vi "FindRequestBySummary.vi"(8 "error in (no error)":errorcluster, 10 "Request Summary":string, 11 "Requests":refnum<class "Request.lvclass">[](array[class])) -> (0 "error out":errorcluster, 1 "Index":i32, 2 "Request out":refnum<class "Request.lvclass">, 3 "Requests out":refnum<class "Request.lvclass">[](array[class]))   [LabVIEW 2015]
uses:
  LVClasses/Request/Request.lvclass
  LVClasses/Request/Request.lvclass/Request.ctl
  <vilib>/Utility/error.llb/Error Cluster From Error Code.vi
  <vilib>/ErrorRing/Error Ring.xnode
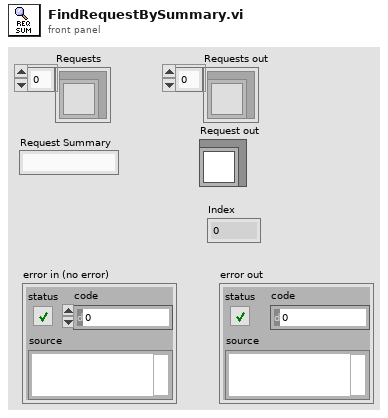
[diagram p1: front panel]
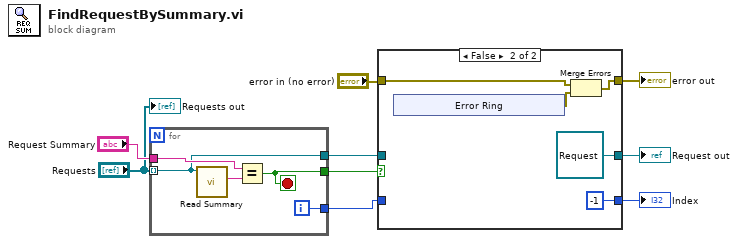
[diagram p0: block diagram]
diagram:
  n1 = for {
    tunnel: "Requests" -> [w10] mode=indexing
    tunnel: "Request Summary" -> [w13]
    tunnel: [w12] -> w3
    tunnel: [w11] -> w5
    tunnel: [w10] -> w6
    i -> [w11]
    stop <- w12 stop-if-true
    n2 = call "Read Summary.vi"("Request in"=w10) -> ("Description"=w14:string)  [unwired: 8 in, 2 out]
    n3 = Equal?(x=w13, y=w14) -> (x = y?=w12:bool)
  }
  n4 = case shown="False" w3 {
    tunnel: [w16 -1] -> w4
    tunnel: w5 -> [w16 _]
    tunnel: w6 -> [w17 _]
    tunnel: [w17 refnum<class "Request.lvclass"> refnum ("Request out")] -> w7
    tunnel: [w15 w18] -> w8
    tunnel: "error in (no error)" -> [w15 w19]
    frame True {
    }
    frame False {
      n5 = xnode "Error Ring"() -> ("error out"=w20:errorcluster)
      n6 = Merge Errors(w19, w20) -> (w18:errorcluster)
    }
  }
  "Index" <- w4
  "Request out" <- w7
  "error out" <- w8
  "Requests out" <- "Requests"
